vi "ConvolveFRF.vi"(8 "musical piece":waveform(dbl)[](graph)=[{"t0"=timestamp(0 s since 1904-01-01), "dt"=2.0833333333333333e-05, "Y"=array[288010 elements]}, {"t0"=timestamp(0 s since 1904-01-01), "dt"=2.0833333333333333e-05, "Y"=array[288010 elements]}], 9 "Sampling rate":u16=48000, 11 "Complex FRF":cluster{"t0":dbl, "dt":dbl, "Y":cdb[]}) -> (0 "Re":T1(graph), 1 "Im":T1(graph), 3 "Convolution":waveform(dbl)(graph), 4 "ratio":dbl format="%0.2e")   [LabVIEW 2022 SP3]
uses:
  <vilib>/Analysis/NI_AALPro.lvlib
  <vilib>/Analysis/NI_AALBase.lvlib
  <vilib>/measure/NI_MAPro.lvlib
  <vilib>/measure/maresamp.llb/Resample Waveform (single shot).vi
  <vilib>/Analysis/2dsp.llb/1D Convolution (DBL).vi
  <vilib>/Analysis/2dsp.llb/Inverse Complex FFT.vi
  <vilib>/Analysis/5stat.llb/RMS (DBL).vi
panel:
  out "1/x":dbl
  out "long time rms":dbl format="%0.2e"
  out "starting rms":dbl format="%0.2f"
  in  "Full?":bool
  out "Waveform Graph 4":cluster{"index":i32, dbl, "X":dbl[]}(graph)
  out "FRF":cluster{"t0":dbl, "dt":dbl, "Y":dbl[]}(graph)
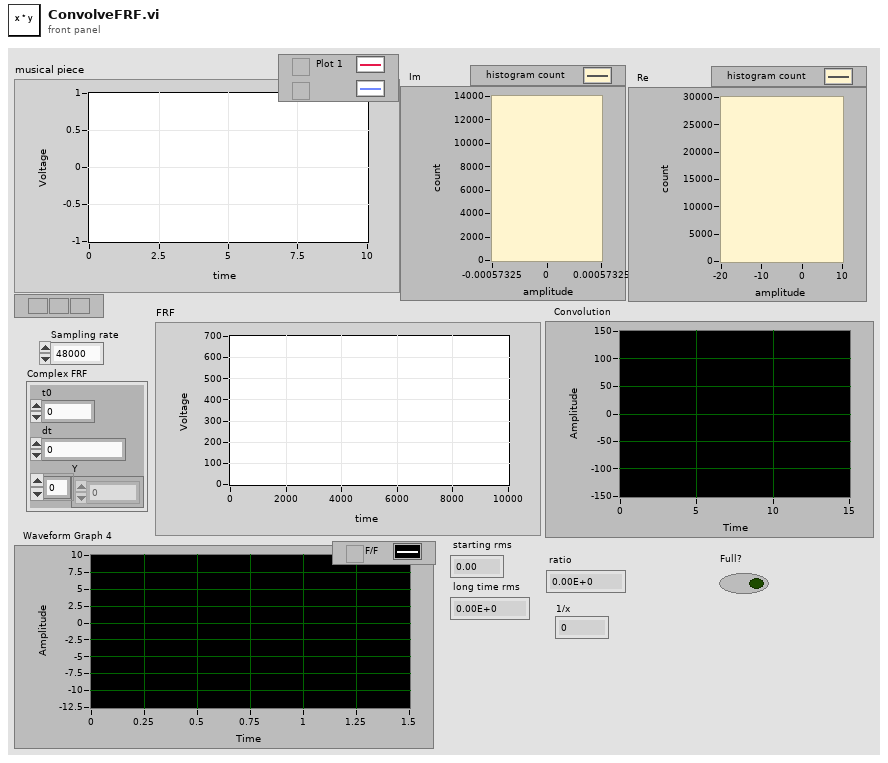
[diagram p1: front panel]
types:
  T1 = cluster{"X Values":dbl[], "Histogram: h(x)":i32[]}
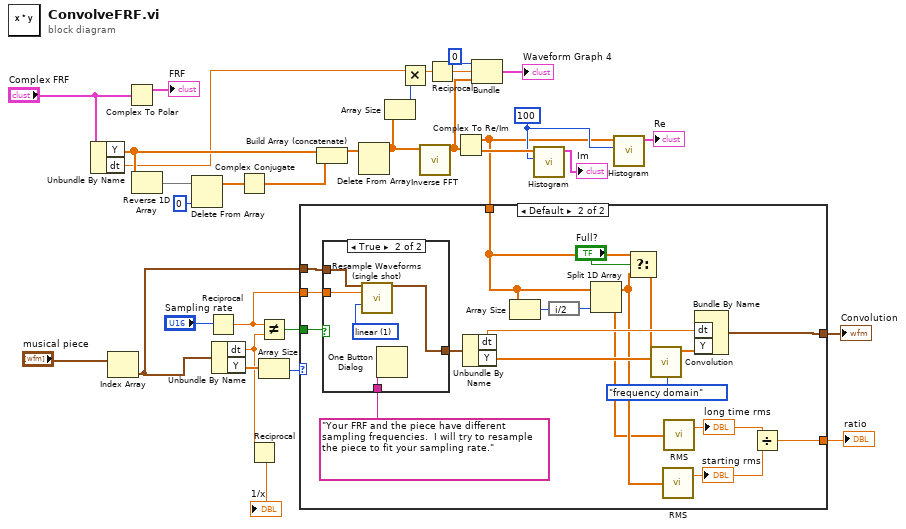
[diagram p0: block diagram]
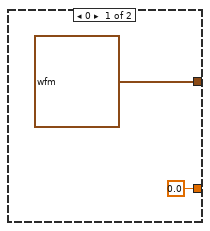
[diagram p2: hidden frame]
diagram:
  w29 = 100 ("intervals")
  n1 = Unbundle By Name("Complex FRF") -> ("Y"=w20:cdb[], "dt"=w10:dbl)
  n2 = Index Array(array="musical piece") -> (element=w16:waveform(dbl))  [unwired: 1 in]
  n3 = Complex To Polar(r * e^(i*theta)="Complex FRF") -> (r=→"FRF":cluster{"t0":dbl, "dt":dbl, "Y":dbl[]})  [unwired: 1 out]
  n4 = Reverse 1D Array(array=w20) -> (reversed array=w31:cdb[])
  n5 = Delete From Array(array=w31, index=0) -> (array with subset deleted=w18:cdb[])  [unwired: 1 in, 1 out]
  n6 = Reciprocal(x="Sampling rate") -> (1/x=w22:dbl)
  n7 = Unbundle By Name(w16) -> ("dt"=w2:dbl, "Y"=w14:dbl[])
  n8 = Complex Conjugate(1:w18) -> (0:w17:cdb[])
  n9 = Reciprocal(x=w2) -> (1/x=→"1/x":dbl)
  n10 = Not Equal?(x=w22, y=w2) -> (x != y?=w26:bool)
  n11 = Array Size(array=w14) -> (size(s)=w13:i32)
  n12 = Build Array (concatenate)(w20, w17) -> (w21:cdb[])
  n13 = Delete From Array(array=w21) -> (array with subset deleted=w9:cdb[])  [unwired: 2 in, 1 out]
  n14 = Array Size(array=w9) -> (size(s)=w8:i32)
  n15 = Multiply(x=w10, y=w8) -> (x*y=w7:dbl)
  n16 = call-poly <vilib>:"Inverse FFT.vi"("FFT {X}"=w9) -> ("X"=w6:cdb[])  [unwired: 9 in, 1 out]
  n17 = Reciprocal(x=w7) -> (1/x=w3:dbl)
  n18 = Complex To Re/Im(x + iy=w6) -> (x=w12:dbl[], y=w30:dbl[])
  n19 = case shown="Default" w13 {
    tunnel: w26 -> [_ w52]
    tunnel: w22 -> [_ w48]
    tunnel: w12 -> [_ w44]
    tunnel: [waveform(dbl) {"t0"=timestamp(0 s since 1904-01-01), "dt"=1.0, "Y"=[]} w42] -> w19
    tunnel: w16 -> [_ w40]
    tunnel: [0.0 w35] -> w11
    frame 0 {
    }
    frame Default {
      n20 = case shown="True" w52 {
        tunnel: "Your FRF and the piece have different sampling frequencies.  I will try to resample the piece to fit your sampling rate." ("message") -> [_ w60]
        tunnel: w40 -> [w55 w59]
        tunnel: [w55 w57] -> w50
        tunnel: w48 -> [_ w56]
        frame False {
        }
        frame True {
          w58 = u16 1 items=["coerce", "linear", "spline", "FIR filter"] ("interpolation mode")
          n21 = call-poly <vilib>:"Resample Waveforms (single shot).vi"("waveform in"=w59, "dt"=w56, "interpolation mode"=w58) -> ("resampled waveform out"=w57:waveform(dbl))  [unwired: 9 in, 3 out]
          n22 = One Button Dialog(message=w60) -> ()  [unwired: 1 in, 1 out]
        }
      }
      n23 = Unbundle By Name(w50) -> ("dt"=w49:dbl, "Y"=w41:dbl[])
      n24 = Array Size(array=w44) -> (size(s)=w47:i32)
      n25 = expression code="i/2"(w47) -> (w46:i32)
      n26 = Split 1D Array(array=w44, index=w46) -> (first subarray=w39:dbl[], second subarray=w38:dbl[])
      n27 = Select(t=w44, s="Full?", f=w39) -> (s? t:f=w43:dbl[])
      n28 = call-poly <vilib>:"Convolution.vi"("algorithm"=enum32{"direct", "frequency domain"}."frequency domain", "Y"=w41, "X"=w43) -> ("X * Y"=w53:dbl[])  [unwired: 7 in, 1 out]
      n29 = call-poly <vilib>:"RMS.vi"("X"=w39) -> ("rms value"=w37:dbl)  [unwired: 1 out]
      "starting rms" <- w37
      n30 = call-poly <vilib>:"RMS.vi"("X"=w38) -> ("rms value"=w36:dbl)  [unwired: 1 out]
      "long time rms" <- w36
      n31 = Bundle By Name("dt"=w49, "Y"=w53) -> (w42:waveform(dbl))  [unwired: 1 in]
      n32 = Divide(x=w36, y=w37) -> (x/y=w35:dbl)
    }
  }
  "Convolution" <- w19
  "ratio" <- w11
  n33 = Bundle("index"=0, w3, "X"=w6) -> (→"Waveform Graph 4":cluster{"index":i32, dbl, "X":cdb[]})  [unwired: 1 in]
  n34 = call <vilib>:"Histogram.vi"("intervals"=w29, "X"=w30) -> ("Histogram Graph"=→"Im":T1)  [unwired: 6 in, 3 out]
  n35 = call <vilib>:"Histogram.vi"("intervals"=w29, "X"=w12) -> ("Histogram Graph"=→"Re":T1)  [unwired: 6 in, 3 out]
